vi "获取量程参数存入关键参数.vi"(8 "error in (no error)":errorcluster caption="错误输入（无错误）", 9 "量程":u16, 10 "flowid":u16, 11 "id":u16) -> (0 "error out":errorcluster caption="错误输出")   [LabVIEW 2016, in "斯坦道CODcr.lvlib"]
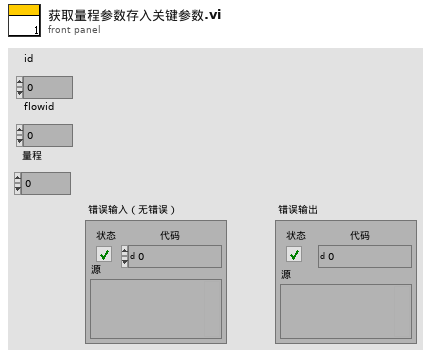
[diagram p1: front panel]
types:
  T1 = cluster{"运行模式":enum16{"维护模式", "常规模式", "应急模式", "质控模式"}, "质控频次":enum16{"关闭", "每天", "星期一", "星期二", "星期三", "星期四", "星期五", "星期六", "星期日"}, "空白核查时间":u16, "跨度核查时间":u16, "测量间隔":u16}
  T2 = cluster{"标液浓度1":dbl, "测量吸光度1":dbl, "样品1启用":bool, "标液浓度2":dbl, "测量吸光度2":dbl, "样品2启用":bool, "标液浓度3":dbl, "测量吸光度3":dbl, "样品3启用":bool, "标液浓度4":dbl, "测量吸光度4":dbl, "样品4启用":bool, "标液浓度5":dbl, "测量吸光度5":dbl, "样品5启用":bool, "模型":enum32{"线性", "多项式"}, "精度":dbl, "XY图":cluster{"X Values":dbl[], "Y Values":dbl[]}[], "拟合公式":string, "r^2":dbl, "标样一校准时间":timestamp, "标样二校准时间":timestamp, "标样三校准时间":timestamp, "标样四校准时间":timestamp, "标样五校准时间":timestamp, "二次方程":cluster{"c":dbl, "x":dbl, "x^2":dbl}, "标定时间":timestamp}
  T3 = cluster{"测量精度":u16, "检出限":dbl, "上限":dbl, "下限":dbl, "阈值（低->高）":dbl, "阈值（高->低）":dbl, "稀释度":dbl}
  T4 = cluster{"泵类型":u8, "进样速度":u32, "出样速度":u32, "泵阀量":u8, "光谱仪类型":u8, "光谱采样次数":u8, "氙灯次数":u8, "B":u16, "C":u16, "D":u16, "E":u16, "B_COD":u16, "C_COD":u16, "D_COD":u16, "E_COD":u16, "G":u16, "M":u16, "N":u16, "氨氮注射泵控温下限":sgl, "氨氮注射泵控温上限":sgl, "总氮注射泵控温下限":sgl, "总氮注射泵控温上限":sgl, "消解温度下限":sgl, "消解温度上限":sgl, "加热10s限值":sgl, "高温高压阀开阀温度":sgl, "总氮x公式0":u8, "总氮x公式1":sgl, "总氮x公式2":sgl, "总磷浊度稀释系数":sgl, "总磷浊度补偿权重1":sgl, "总磷浊度补偿权重2":sgl, "盐度系数":sgl, "氨氮补偿系数1":sgl, "氨氮补偿系数2":sgl}
  T5 = cluster{"标液浓度1":dbl, "测量吸光度1":dbl, "样品1启用":bool, "标液浓度2":dbl, "测量吸光度2":dbl, "样品2启用":bool, "标液浓度3":dbl, "测量吸光度3":dbl, "样品3启用":bool, "标液浓度4":dbl, "测量吸光度4":dbl, "样品4启用":bool, "标液浓度5":dbl, "测量吸光度5":dbl, "样品5启用":bool, "模型":enum32{"线性", "多项式"}, "精度":dbl, "XY图":cluster{"X Values":dbl[], "Y Values":dbl[]}[], "拟合公式":string, "r^2":dbl, "标样一校准时间":timestamp, "标样二校准时间":timestamp, "标样三校准时间":timestamp, "标样四校准时间":timestamp, "标样五校准时间":timestamp, "二次方程":cluster{"c":dbl, "x":dbl, "x^2":dbl}, "标定时间":timestamp}[]
  T6 = typedef "斯坦道CODcr.lvlib/关键参数.ctl" = cluster{"测量量程":sgl, "测量检出限":sgl, "测量精度":sgl, "测量间隔":sgl, "消解温度":sgl, "消解时长":sgl, "三项式系数":sgl, "二次多项式系数":sgl, "曲线斜率":sgl, "曲线截距":sgl, "线性相关系数":sgl, "空白校准时间":timestamp, "标样校准时间":timestamp, "测量信号值":sgl, "稀释倍数":sgl, "空白标定系数":sgl, "量程系数":sgl}
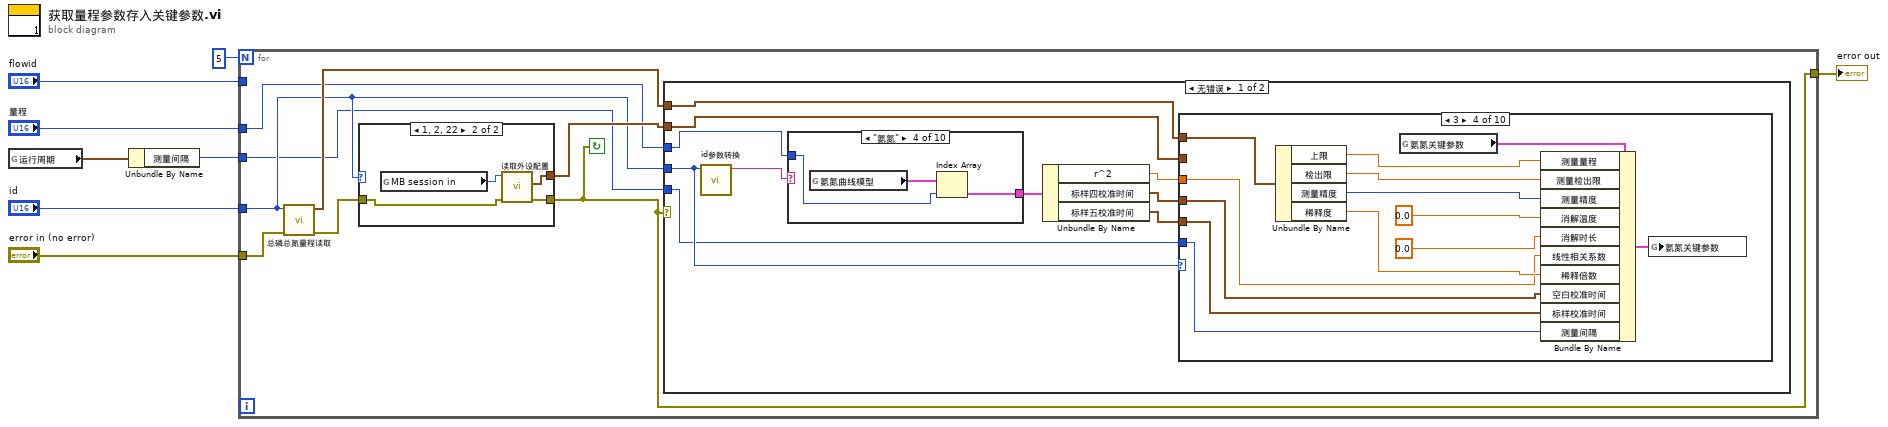
[diagram p0: block diagram]
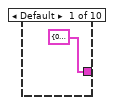
[diagram p3: hidden frame]
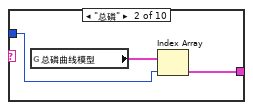
[diagram p4: hidden frame]
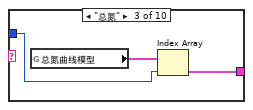
[diagram p5: hidden frame]
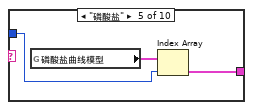
[diagram p6: hidden frame]
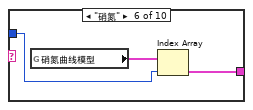
[diagram p7: hidden frame]
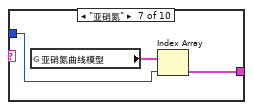
[diagram p8: hidden frame]
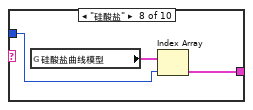
[diagram p9: hidden frame]
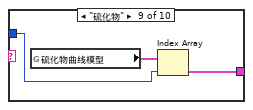
[diagram p10: hidden frame]
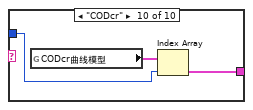
[diagram p11: hidden frame]
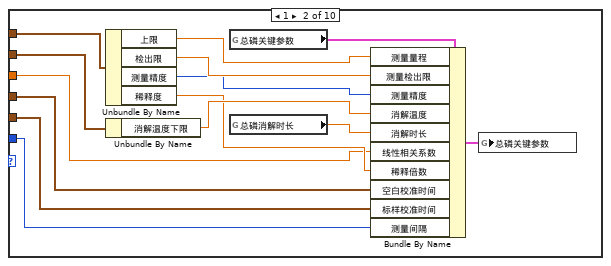
[diagram p13: hidden frame]
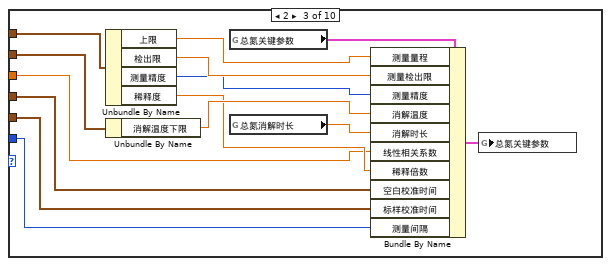
[diagram p14: hidden frame]
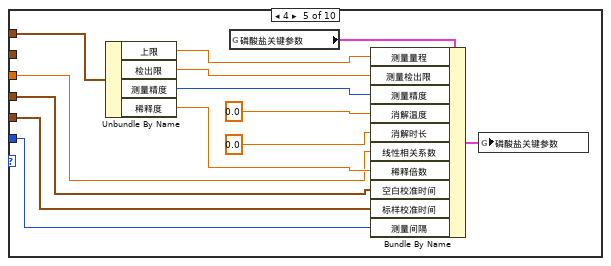
[diagram p15: hidden frame]
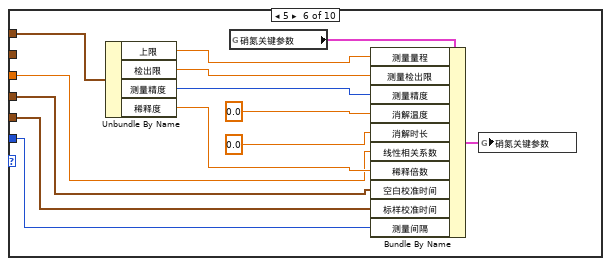
[diagram p16: hidden frame]
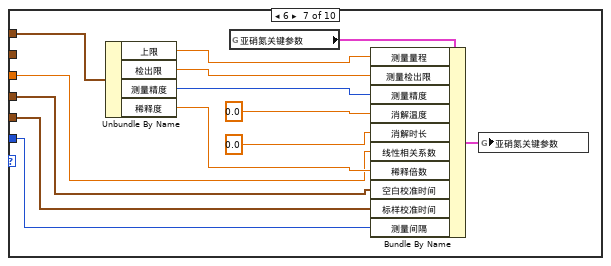
[diagram p17: hidden frame]
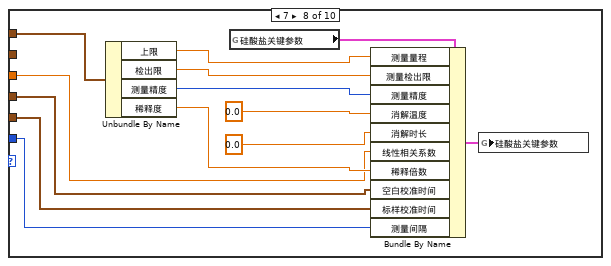
[diagram p18: hidden frame]
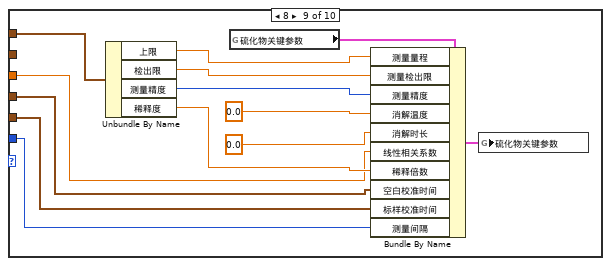
[diagram p19: hidden frame]
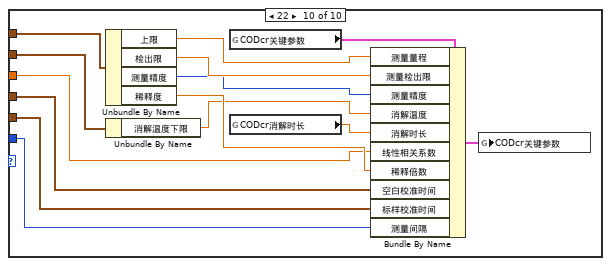
[diagram p20: hidden frame]
diagram:
  n1 = global read "总磷总氮断电保存全局变量.vi" "运行周期"() -> (w2:T1)
  n2 = Unbundle By Name(w2) -> ("测量间隔"=w1:u16)
  n3 = for {
    N: 5 -> [_]
    tunnel: "量程" -> [w14]
    tunnel: "flowid" -> [_]
    tunnel: "id" -> [w10]
    tunnel: "error in (no error)" -> [w11]
    tunnel: [w12] -> w3
    tunnel: w1 -> [w9]
    stop <- w12 continue-if-true
    n4 = call "总磷总氮量程读取.vi"("error in (no error)"=w11, "测量参数"=w10) -> ("error out"=w13:errorcluster, "量程参数读取"=w16:T3)  [unwired: 8 in]
    n5 = case shown="1, 2, 22" w10 {
      tunnel: [_ w20] -> w15
      tunnel: w13 -> [w17 w19]
      tunnel: [w17 w18] -> w12
      frame 0, Default {
      }
      frame 1, 2, 22 {
        n6 = global read "VAR总磷总氮全局变量.vi" "MB session in"() -> (w21:refnum<class "MB_Master.lvclass">)
        n7 = call "读取外设配置.vi"("error in (no error)"=w19, "MB session in"=w21) -> ("error out"=w18:errorcluster, "外设配置"=w20:T4)  [unwired: 7 in, 1 out]
      }
    }
    n8 = case shown="无错误" w12 {
      tunnel: w16 -> [w31 _]
      tunnel: w15 -> [w30 _]
      tunnel: w10 -> [w23 _]
      tunnel: w14 -> [w24 _]
      tunnel: w9 -> [w22 _]
      frame No Error {
        n9 = call "id参数转换.vi"("id"=w23) -> ("table输出"=w29:string)  [unwired: 9 in, 1 out]
        n10 = case shown="\"氨氮\"" w29 {
          tunnel: w24 -> [_ w33 w36 w39 w42 w45 w48 w51 w54 w57]
          tunnel: [T2 {"标液浓度1"=0.0, "测量吸光度1"=0.0, "样品1启用"=FALSE, "标液浓度2"=0.0, "测量吸光度2"=0.0, "样品2启用"=FALSE, "标液浓度3"=0.0, "测量吸光度3"=0.0, "样品3启用"=FALSE, "标液浓度4"=0.0, "测量吸光度4"=0.0, "样品4启用"=FALSE, "标液浓度5"=0.0, "测量吸光度5"=0.0, "样品5启用"=FALSE, "模型"=enum."线性", "精度"=0.0, "XY图"=[], "拟合公式"="", "r^2"=0.0, "标样一校准时间"=timestamp(0 s since 1904-01-01), "标样二校准时间"=timestamp(0 s since 1904-01-01), "标样三校准时间"=timestamp(0 s since 1904-01-01), "标样四校准时间"=timestamp(0 s since 1904-01-01), "标样五校准时间"=timestamp(0 s since 1904-01-01), "二次方程"={"c"=0.0, "x"=0.0, "x^2"=0.0}, "标定时间"=timestamp(0 s since 1904-01-01)} ("总磷曲线模型") w34 w37 w40 w43 w46 w49 w52 w55 w58] -> w28
          frame Default {
          }
          frame "总磷" {
            n11 = global read "校准数据全局变量.vi" "总磷曲线模型"() -> (w35:T5)
            n12 = Index Array(array=w35, index=w33) -> (element=w34:T2)
          }
          frame "总氮" {
            n13 = global read "校准数据全局变量.vi" "总氮曲线模型"() -> (w38:T5)
            n14 = Index Array(array=w38, index=w36) -> (element=w37:T2)
          }
          frame "氨氮" {
            n15 = global read "校准数据全局变量.vi" "氨氮曲线模型"() -> (w41:T5)
            n16 = Index Array(array=w41, index=w39) -> (element=w40:T2)
          }
          frame "磷酸盐" {
            n17 = global read "校准数据全局变量.vi" "磷酸盐曲线模型"() -> (w44:T5)
            n18 = Index Array(array=w44, index=w42) -> (element=w43:T2)
          }
          frame "硝氮" {
            n19 = global read "校准数据全局变量.vi" "硝氮曲线模型"() -> (w47:T5)
            n20 = Index Array(array=w47, index=w45) -> (element=w46:T2)
          }
          frame "亚硝氮" {
            n21 = global read "校准数据全局变量.vi" "亚硝氮曲线模型"() -> (w50:T5)
            n22 = Index Array(array=w50, index=w48) -> (element=w49:T2)
          }
          frame "硅酸盐" {
            n23 = global read "校准数据全局变量.vi" "硅酸盐曲线模型"() -> (w53:T5)
            n24 = Index Array(array=w53, index=w51) -> (element=w52:T2)
          }
          frame "硫化物" {
            n25 = global read "校准数据全局变量.vi" "硫化物曲线模型"() -> (w56:T5)
            n26 = Index Array(array=w56, index=w54) -> (element=w55:T2)
          }
          frame "CODcr" {
            n27 = global read "校准数据全局变量.vi" "CODcr曲线模型"() -> (w59:T5)
            n28 = Index Array(array=w59, index=w57) -> (element=w58:T2)
          }
        }
        n29 = Unbundle By Name(w28) -> ("r^2"=w27:dbl, "标样四校准时间"=w26:timestamp, "标样五校准时间"=w25:timestamp)
        n30 = case shown="3" w23 {
          tunnel: w31 -> [_ w71 w85 w98 w111 w124 w137 w150 w163 w177]
          tunnel: w30 -> [_ w67 w81 _ _ _ _ _ _ w172]
          tunnel: w27 -> [_ w61 w77 w91 w102 w117 w130 w143 w154 w169]
          tunnel: w26 -> [_ w62 w76 w90 w104 w116 w129 w142 w156 w168]
          tunnel: w25 -> [_ w63 w75 w89 w103 w115 w128 w141 w155 w167]
          tunnel: w22 -> [_ w60 w74 w88 w101 w114 w127 w140 w153 w166]
          frame 0, Default {
          }
          frame 1 {
            n31 = Unbundle By Name(w71) -> ("上限"=w70:dbl, "检出限"=w69:dbl, "测量精度"=w68:u16, "稀释度"=w64:dbl)
            n32 = Unbundle By Name(w67) -> ("消解温度下限"=w66:sgl)
            n33 = global read "VAR总磷总氮全局变量.vi" "总磷关键参数"() -> (w72:T6)
            n34 = global read "总磷总氮断电保存全局变量.vi" "总磷消解时长"() -> (w65:dbl)
            n35 = Bundle By Name(cluster=w72, "测量量程"=w70, "测量检出限"=w69, "测量精度"=w68, "消解温度"=w66, "消解时长"=w65, "线性相关系数"=w61, "稀释倍数"=w64, "空白校准时间"=w62, "标样校准时间"=w63, "测量间隔"=w60) -> (w73:T6)
            n36 = global write "VAR总磷总氮全局变量.vi" "总磷关键参数"(w73) -> ()
          }
          frame 2 {
            n37 = Unbundle By Name(w85) -> ("上限"=w84:dbl, "检出限"=w83:dbl, "测量精度"=w82:u16, "稀释度"=w78:dbl)
            n38 = Unbundle By Name(w81) -> ("消解温度下限"=w80:sgl)
            n39 = global read "VAR总磷总氮全局变量.vi" "总氮关键参数"() -> (w86:T6)
            n40 = global read "总磷总氮断电保存全局变量.vi" "总氮消解时长"() -> (w79:dbl)
            n41 = Bundle By Name(cluster=w86, "测量量程"=w84, "测量检出限"=w83, "测量精度"=w82, "消解温度"=w80, "消解时长"=w79, "线性相关系数"=w77, "稀释倍数"=w78, "空白校准时间"=w76, "标样校准时间"=w75, "测量间隔"=w74) -> (w87:T6)
            n42 = global write "VAR总磷总氮全局变量.vi" "总氮关键参数"(w87) -> ()
          }
          frame 3 {
            n43 = Unbundle By Name(w98) -> ("上限"=w97:dbl, "检出限"=w96:dbl, "测量精度"=w95:u16, "稀释度"=w94:dbl)
            n44 = global read "VAR总磷总氮全局变量.vi" "氨氮关键参数"() -> (w99:T6)
            n45 = Bundle By Name(cluster=w99, "测量量程"=w97, "测量检出限"=w96, "测量精度"=w95, "消解温度"=sgl 0.0, "消解时长"=sgl 0.0, "线性相关系数"=w91, "稀释倍数"=w94, "空白校准时间"=w90, "标样校准时间"=w89, "测量间隔"=w88) -> (w100:T6)
            n46 = global write "VAR总磷总氮全局变量.vi" "氨氮关键参数"(w100) -> ()
          }
          frame 4 {
            n47 = Unbundle By Name(w111) -> ("上限"=w110:dbl, "检出限"=w109:dbl, "测量精度"=w108:u16, "稀释度"=w107:dbl)
            n48 = global read "VAR总磷总氮全局变量.vi" "磷酸盐关键参数"() -> (w112:T6)
            n49 = Bundle By Name(cluster=w112, "测量量程"=w110, "测量检出限"=w109, "测量精度"=w108, "消解温度"=sgl 0.0, "消解时长"=sgl 0.0, "线性相关系数"=w102, "稀释倍数"=w107, "空白校准时间"=w104, "标样校准时间"=w103, "测量间隔"=w101) -> (w113:T6)
            n50 = global write "VAR总磷总氮全局变量.vi" "磷酸盐关键参数"(w113) -> ()
          }
          frame 5 {
            n51 = Unbundle By Name(w124) -> ("上限"=w123:dbl, "检出限"=w122:dbl, "测量精度"=w121:u16, "稀释度"=w120:dbl)
            n52 = global read "VAR总磷总氮全局变量.vi" "硝氮关键参数"() -> (w125:T6)
            n53 = Bundle By Name(cluster=w125, "测量量程"=w123, "测量检出限"=w122, "测量精度"=w121, "消解温度"=sgl 0.0, "消解时长"=sgl 0.0, "线性相关系数"=w117, "稀释倍数"=w120, "空白校准时间"=w116, "标样校准时间"=w115, "测量间隔"=w114) -> (w126:T6)
            n54 = global write "VAR总磷总氮全局变量.vi" "硝氮关键参数"(w126) -> ()
          }
          frame 6 {
            n55 = Unbundle By Name(w137) -> ("上限"=w136:dbl, "检出限"=w135:dbl, "测量精度"=w134:u16, "稀释度"=w133:dbl)
            n56 = global read "VAR总磷总氮全局变量.vi" "亚硝氮关键参数"() -> (w138:T6)
            n57 = Bundle By Name(cluster=w138, "测量量程"=w136, "测量检出限"=w135, "测量精度"=w134, "消解温度"=sgl 0.0, "消解时长"=sgl 0.0, "线性相关系数"=w130, "稀释倍数"=w133, "空白校准时间"=w129, "标样校准时间"=w128, "测量间隔"=w127) -> (w139:T6)
            n58 = global write "VAR总磷总氮全局变量.vi" "亚硝氮关键参数"(w139) -> ()
          }
          frame 7 {
            n59 = Unbundle By Name(w150) -> ("上限"=w149:dbl, "检出限"=w148:dbl, "测量精度"=w147:u16, "稀释度"=w146:dbl)
            n60 = global read "VAR总磷总氮全局变量.vi" "硅酸盐关键参数"() -> (w151:T6)
            n61 = Bundle By Name(cluster=w151, "测量量程"=w149, "测量检出限"=w148, "测量精度"=w147, "消解温度"=sgl 0.0, "消解时长"=sgl 0.0, "线性相关系数"=w143, "稀释倍数"=w146, "空白校准时间"=w142, "标样校准时间"=w141, "测量间隔"=w140) -> (w152:T6)
            n62 = global write "VAR总磷总氮全局变量.vi" "硅酸盐关键参数"(w152) -> ()
          }
          frame 8 {
            n63 = Unbundle By Name(w163) -> ("上限"=w162:dbl, "检出限"=w161:dbl, "测量精度"=w160:u16, "稀释度"=w159:dbl)
            n64 = global read "VAR总磷总氮全局变量.vi" "硫化物关键参数"() -> (w164:T6)
            n65 = Bundle By Name(cluster=w164, "测量量程"=w162, "测量检出限"=w161, "测量精度"=w160, "消解温度"=sgl 0.0, "消解时长"=sgl 0.0, "线性相关系数"=w154, "稀释倍数"=w159, "空白校准时间"=w156, "标样校准时间"=w155, "测量间隔"=w153) -> (w165:T6)
            n66 = global write "VAR总磷总氮全局变量.vi" "硫化物关键参数"(w165) -> ()
          }
          frame 22 {
            n67 = Unbundle By Name(w177) -> ("上限"=w176:dbl, "检出限"=w175:dbl, "测量精度"=w174:u16, "稀释度"=w173:dbl)
            n68 = Unbundle By Name(w172) -> ("消解温度下限"=w171:sgl)
            n69 = global read "VAR总磷总氮全局变量.vi" "CODcr关键参数"() -> (w178:T6)
            n70 = global read "总磷总氮断电保存全局变量.vi" "CODcr消解时长"() -> (w170:dbl)
            n71 = Bundle By Name(cluster=w178, "测量量程"=w176, "测量检出限"=w175, "测量精度"=w174, "消解温度"=w171, "消解时长"=w170, "线性相关系数"=w169, "稀释倍数"=w173, "空白校准时间"=w168, "标样校准时间"=w167, "测量间隔"=w166) -> (w179:T6)
            n72 = global write "VAR总磷总氮全局变量.vi" "CODcr关键参数"(w179) -> ()
          }
        }
      }
      frame Error {
      }
    }
  }
  "error out" <- w3
